vi "Generate write queue item.vi"(8 "error in (no error)":errorcluster, 11 "Goodbye in":refnum<class "Goodbye.lvclass">) -> (0 "error out":errorcluster, 2 "Write queue item":T1, 3 "Goodbye out":refnum<class "Goodbye.lvclass">)   [LabVIEW 2020, in "wamplv.lvlib" / "Goodbye.lvclass"]
uses:
  Goodbye.lvclass
  Goodbye.lvclass/Goodbye.ctl
  TypeDefs/WAMP Message Codes.ctl
  wamplv.lvlib
  b0d296bb-c887-4fa9-b59c-7a0be08ffa36.vi
  TypeDefs/Transport type.ctl
  WAMP Client/Private/TypeDef/Write queue item.ctl
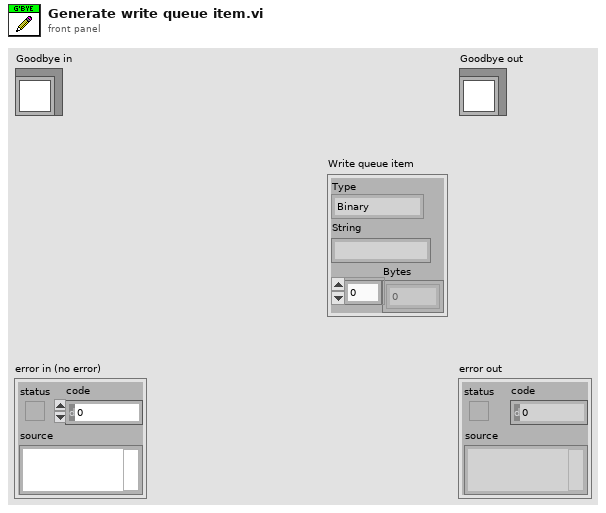
[diagram p1: front panel]
types:
  T1 = typedef "wamplv.lvlib/Write queue item.ctl" = cluster{"Type":T2, "String":string, "Bytes":u8[]}
  T2 = typedef "wamplv.lvlib/Transport type.ctl" = enum16{"Binary", "Text"}
  T3 = typedef "wamplv.lvlib/WAMP Message Codes.ctl" = enum8{"HELLO", "WELCOME", "CHALLENGE", "AUTHENTICATE", "ABORT", "GOODBYE", "ERROR", "PUBLISH", "PUBLISHED", "SUBSCRIBE", "SUBSCRIBED", "UNSUBSCRIBE", "UNSUBSCRIBED", "EVENT", "CALL", "RESULT", "REGISTER", "REGISTERED", "UNREGISTER", "UNREGISTERED", "INVOCATION", "YIELD"}
  T4 = typedef "wamplv.lvlib/WAMP Client.lvclass/Serialisation.ctl" = enum16{"JSON", "MessagePack"}
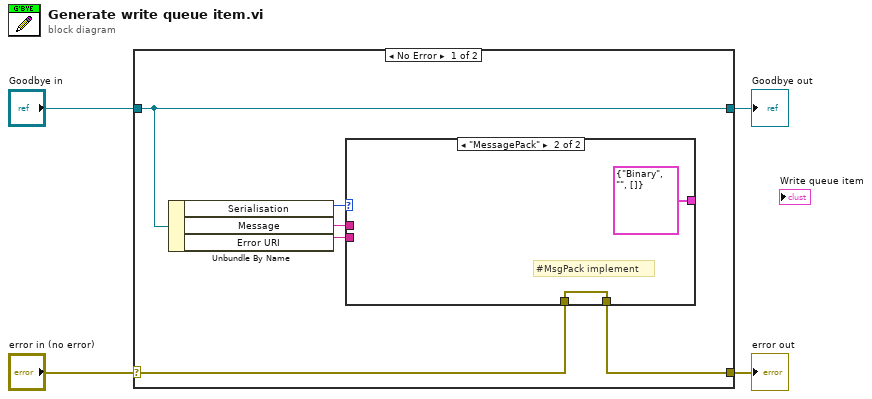
[diagram p0: block diagram]
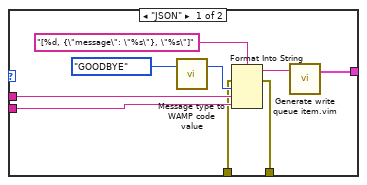
[diagram p2: hidden frame]
diagram:
  n1 = case shown="No Error" "error in (no error)" {
    selector: "error in (no error)" -> [w6 w23]
    tunnel: [w5 w23] -> w3
    tunnel: [w10 w22] -> w1
    tunnel: "Goodbye in" -> [w10 w22]
    frame No Error {
      n2 = Unbundle By Name(w10) -> ("Serialisation"=w9:T4, "Message"=w8:string, "Error URI"=w7:string)
      n3 = case shown="\"MessagePack\"" w9 {
        tunnel: [w16 w20] -> w5
        tunnel: [w14 T1 {"Type"=enum."Binary", "String"="", "Bytes"=[]} ("Ouput")] -> _
        tunnel: w8 -> [w13 _]
        tunnel: w7 -> [w12 _]
        tunnel: w6 -> [w11 w20]
        frame "JSON" {
          n4 = call "Message type to WAMP code value.vi"("Message Type"=WAMP_Message_Codes."GOODBYE" ("Message Codes")) -> ("WAMP Numeric value"=w17:u8)  [unwired: 2 in]
          n5 = Format Into String(format string="[%d, {\"message\": \"%s\"}, \"%s\"]", error in=w11, w17, w13, w12) -> (resulting string=w15:string, error out=w16:errorcluster)  [unwired: 1 in]
          n6 = call "Generate write queue item.vim"("Input"=w15) -> ("Ouput"=w14:T1)  [unwired: 2 in]
        }
        frame "MessagePack" {
          # "#MsgPack implement"
        }
      }
    }
    frame Error {
    }
  }
  "error out" <- w3
  "Goodbye out" <- w1
